vi "Set value.vi"(7 "Ignore range overflow error (false)":bool, 8 "error in":errorcluster, 10 "Value":dbl, 11 "VISA resource name":refnum<visa-resource-name>) -> (0 "error out":errorcluster, 2 "Set value failed":bool, 3 "VISA resource name out":refnum<visa-resource-name>)   [LabVIEW 2013, in "Datron D4xxx.lvlib"]
doc: "This VI sets instrument main register value. Optionaly you can set this VI to ignore main register overflow error (for manual ranges).\nIf function F4 (resistors) is selected, VI sends nearest range or short circuit.\nIf value is not accepted by instrument (for example register overflow) VI returns true at \"Set value failed\" (even if error ignored)."
uses:
  Datron D4xxx.lvlib
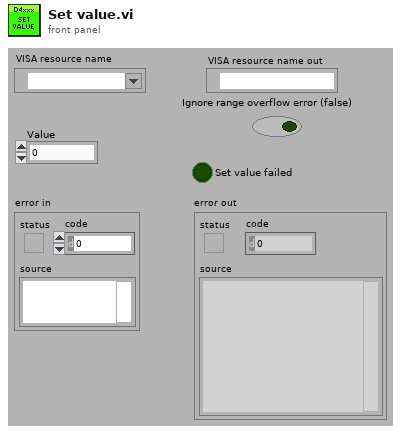
[diagram p1: front panel]
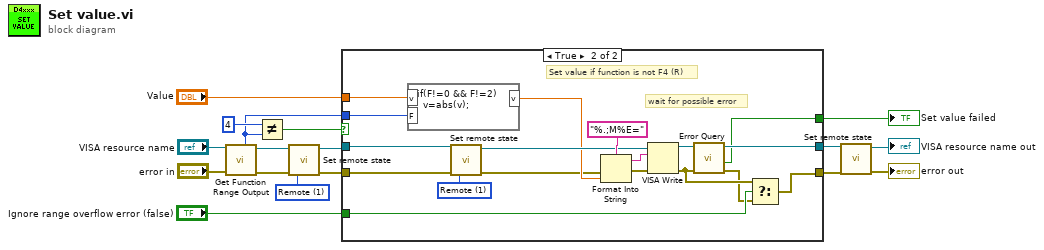
[diagram p0: block diagram]
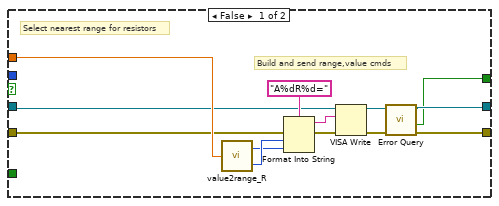
[diagram p2: hidden frame]
diagram:
  w10 = u16 1 items=["Local", "Remote", "Default"] ("Remote state")
  n1 = call "Get Function Range Output.vi"("error in (no error)"="error in", "VISA resource name"="VISA resource name") -> ("error out"=w9:errorcluster, "VISA resource name out"=w7:refnum<visa-resource-name>, "Function {F0-F5}"=w12:i32)  [unwired: 2 in, 5 out]
  n2 = Not Equal?(x=4, y=w12) -> (x != y?=w13:bool)
  n3 = call "Set remote state.vi"("error in"=w9, "Remote state"=w10, "VISA resource name"=w7) -> ("error out"=w8:errorcluster, "VISA resource name out"=w6:refnum<visa-resource-name>)  [unwired: 7 in]
  n4 = case shown="True" w13 {
    tunnel: "Value" -> [w23 w39]
    tunnel: [w20 w32] -> w5
    tunnel: [w19 w33] -> w4
    tunnel: w8 -> [w22 w45]
    tunnel: w6 -> [w21 w44]
    tunnel: w12 -> [_ w40]
    tunnel: "Ignore range overflow error (false)" -> [_ w35]
    tunnel: [w18 w31] -> w1
    frame False {
      # "Build and send range,value cmds"
      # "Select nearest range for resistors"
      n5 = call "value2range_R.vi"("Resistance [Ohm]"=w23) -> ("Nearest range code"=w24:i32, "Zero/full range code"=w25:i32)
      n6 = Format Into String(format string="A%dR%d=", error in=w22, w25, w24) -> (resulting string=w30:string, error out=w29:errorcluster)  [unwired: 1 in]
      n7 = VISA Write(VISA resource name=w21, write buffer=w30, error in (no error)=w29) -> (VISA resource name out=w26:refnum<visa-resource-name>, error out=w27:errorcluster)  [unwired: 1 out]
      n8 = call "Error Query.vi"("error in (no error)"=w27, "VISA resource name"=w26) -> ("error out"=w20:errorcluster, "Error"=w18:bool, "VISA resource name out"=w19:refnum<visa-resource-name>)  [unwired: 6 in, 1 out]
    }
    frame True {
      w42 = u16 1 items=["Local", "Remote", "Default"] ("Remote state")
      # "Set value if function is not F4 (R)"
      # "wait for possible error"
      n9 = formula code="if(F!=0 && F!=2)\n  v=abs(v);"("v"=w39, "F"=w40) -> ("v"=w38:dbl)
      n10 = call "Set remote state.vi"("error in"=w45, "Remote state"=w42, "VISA resource name"=w44) -> ("error out"=w37:errorcluster, "VISA resource name out"=w43:refnum<visa-resource-name>)  [unwired: 7 in]
      n11 = Format Into String(format string="%.;M%E=", error in=w37, w38) -> (resulting string=w48:string, error out=w47:errorcluster)  [unwired: 1 in]
      n12 = VISA Write(VISA resource name=w43, write buffer=w48, error in (no error)=w47) -> (VISA resource name out=w41:refnum<visa-resource-name>, error out=w36:errorcluster)  [unwired: 1 out]
      n13 = call "Error Query.vi"("error in (no error)"=w36, "VISA resource name"=w41) -> ("error out"=w34:errorcluster, "Error"=w31:bool, "VISA resource name out"=w33:refnum<visa-resource-name>)  [unwired: 6 in, 1 out]
      n14 = Select(t=w36, s=w35, f=w34) -> (s? t:f=w32:errorcluster)
    }
  }
  "Set value failed" <- w1
  n15 = call "Set remote state.vi"("error in"=w5, "VISA resource name"=w4) -> ("error out"=→"error out":errorcluster, "VISA resource name out"=→"VISA resource name out":refnum<visa-resource-name>)  [unwired: 8 in]
